vi "compare top countries window.vi"(4 "SA data":T1, 6 "Countries":string[](array[string]), 7 "Aggregate indexes":i32[](array[numeric]), 8 "Populations":i32[](array[numeric]), 9 "US data":T1, 10 "deaths CSV":string[][](array[string]), 11 "cases CSV":string[][](array[string])) -> ()   [LabVIEW 2019]
uses:
  <vilib>/Utility/config.llb/NI_LVConfig.lvlib
panel:
  in  "Tab Control":enum32{"Results", "Filter out"}(tab)
  in  "Include SA provinces":bool
  in  "How far back to look for rate of rise and fall (days)":u16=7
  out "Top cumulative deaths per M":string[](array[string])
  out "Top daily death rate per million ever":string[](array[string])
  out "Top rate of fall in deaths":string[](array[string]) caption="Top rate of fall in deaths (over last 7 days)"
  out "Top rate of rise in deaths (over last 14 days)":string[](array[string]) caption="Top rate of rise in deaths (over last 7 days)"
  out "Top new cases":string[](array[string])
  out "Top new deaths":string[](array[string])
  out "Top new cases per 1M":string[](array[string])
  out "Top new deaths per 1M":string[](array[string])
  in  "Include US states":bool
  in  "Include aggregates":bool
  in  "Aggregates":i32(listbox)
  in  "Remove Button":bool
  in  "Add Button":bool
  in  "Filter out":i32[](listbox)
  in  "Select Country":i32[](listbox)
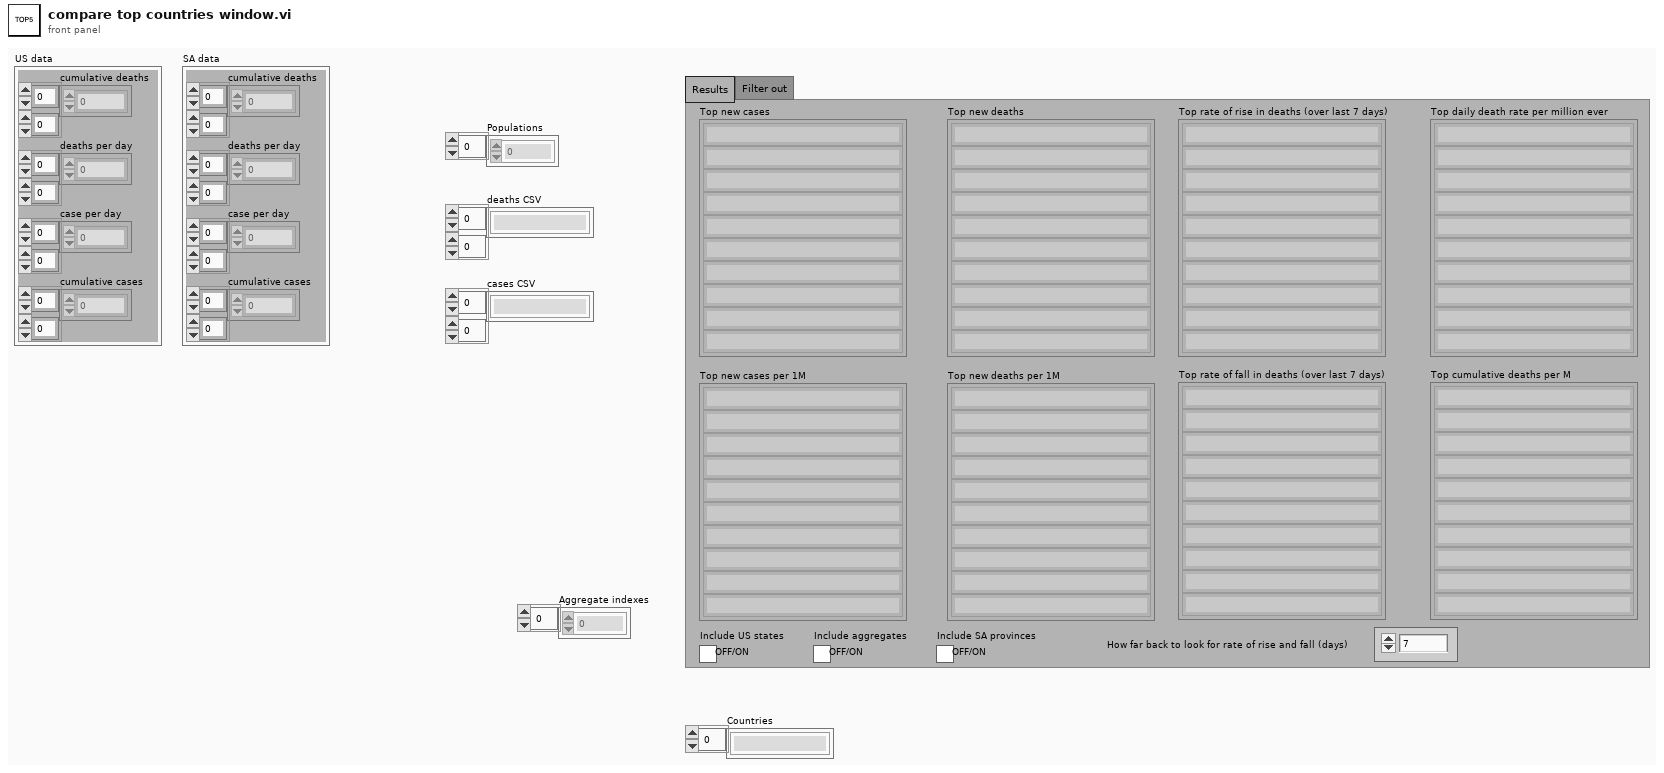
[diagram p1: front panel]
types:
  T1 = cluster{"cumulative deaths":i32[][], "deaths per day":i32[][], "case per day":i32[][], "cumulative cases":i32[][]}
  T2 = typedef "NI_LVConfig.lvlib/Config Data RefNum.ctl" = refnum<k1>
  T3 = cluster{"top new cases":cluster{"country index":i32[], "values":i32[]}, "top new deaths":cluster{"country index":i32[], "values":i32[]}, "top new cases per 1M":cluster{"country index":i32[], "values":dbl[]}, "top new deaths per 1M":cluster{"country index":i32[], "values":dbl[]}, "deaths dropped":cluster{"country index":i32[], "percentage change":dbl[]}, "deaths gained":cluster{"country index":i32[], "percentage change":dbl[]}, "highest deaths per day ever":cluster{"country index":i32[], "highest deaths per day":dbl[]}, "highest deaths":cluster{"country index":i32[], "highest deaths per day":dbl[]}}
  T4 = cluster{"country index":i32[], "percentage change":dbl[]}
  T5 = cluster{"country index":i32[], "highest deaths per day":dbl[]}
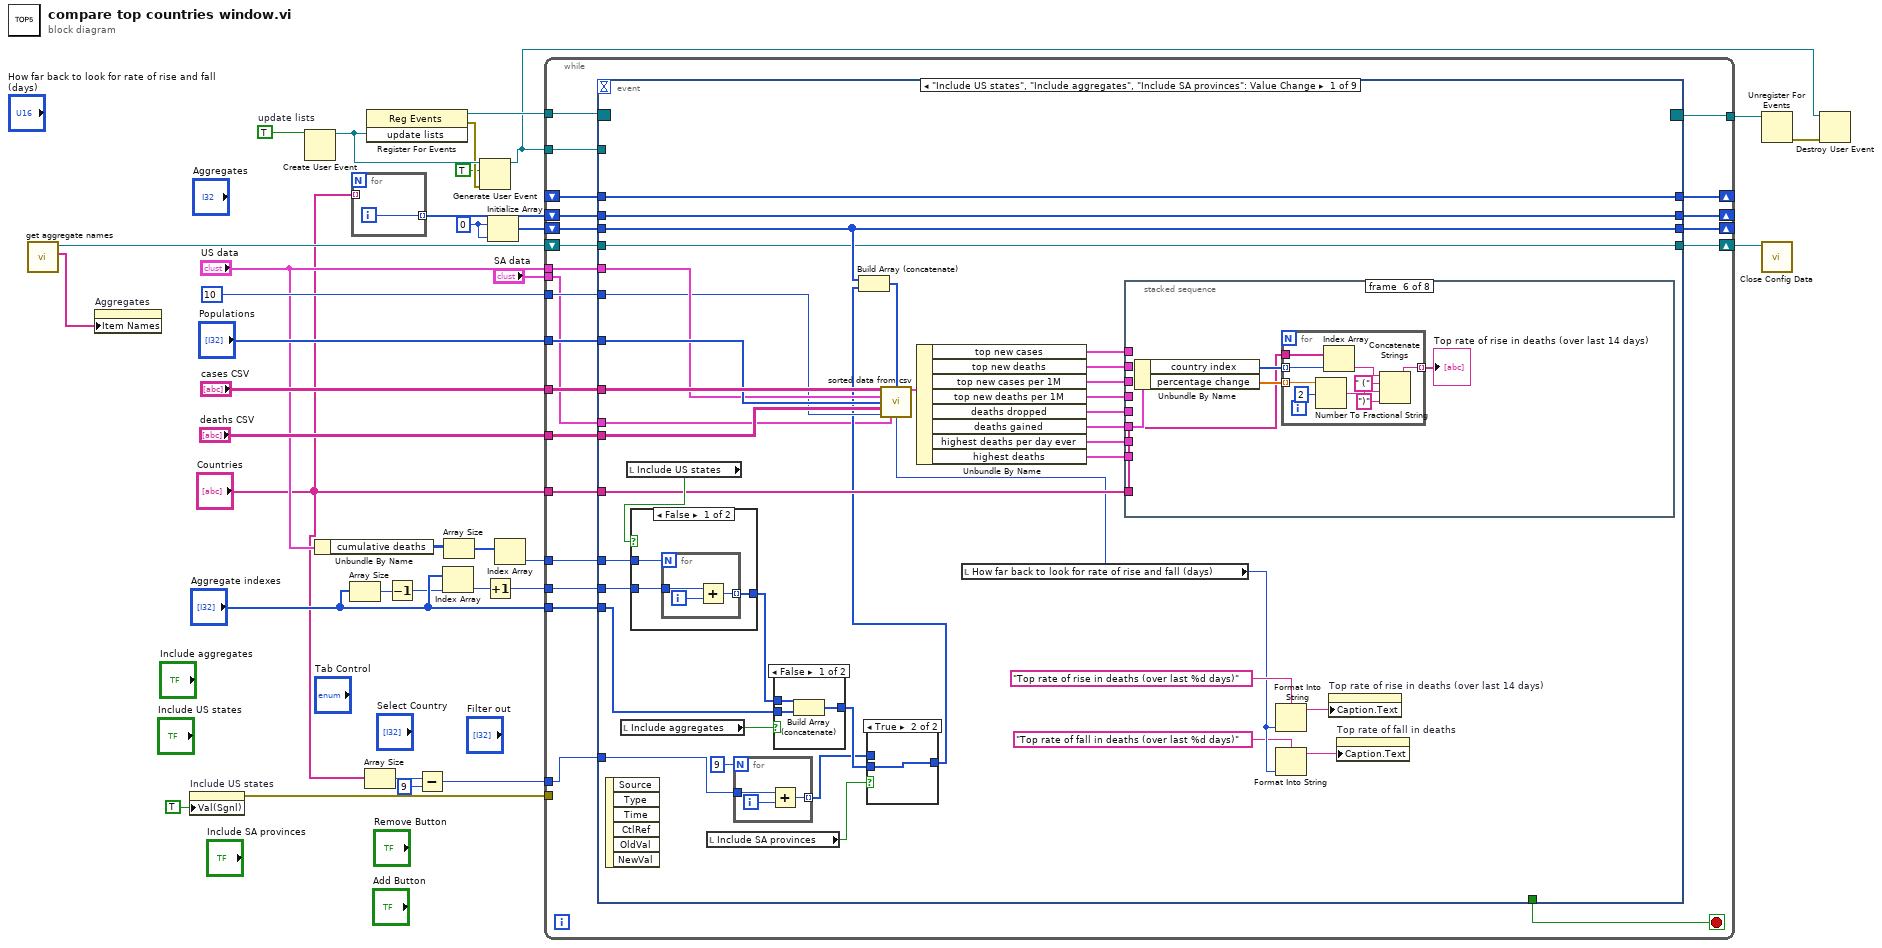
[diagram p0: block diagram]
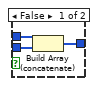
[diagram p2: hidden frame]
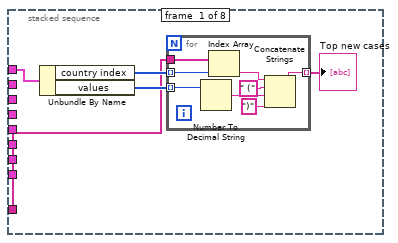
[diagram p3: hidden frame]
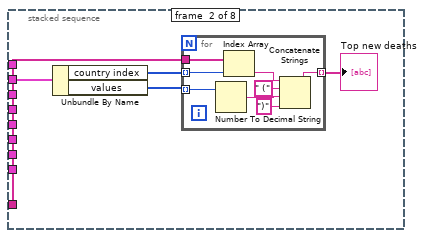
[diagram p4: hidden frame]
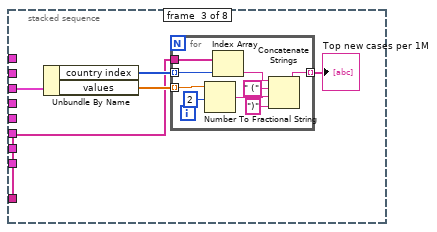
[diagram p5: hidden frame]
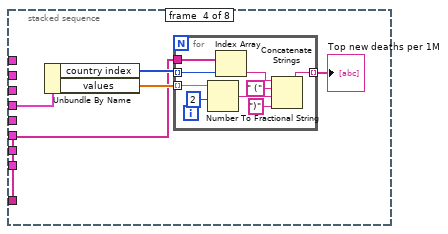
[diagram p6: hidden frame]
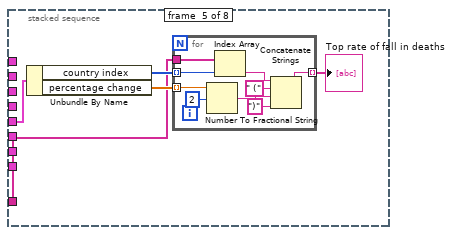
[diagram p7: hidden frame]
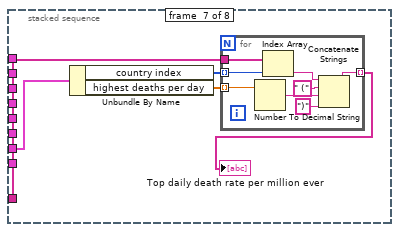
[diagram p8: hidden frame]
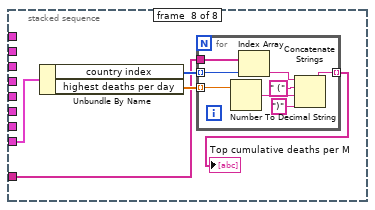
[diagram p9: hidden frame]
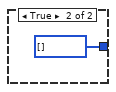
[diagram p10: hidden frame]
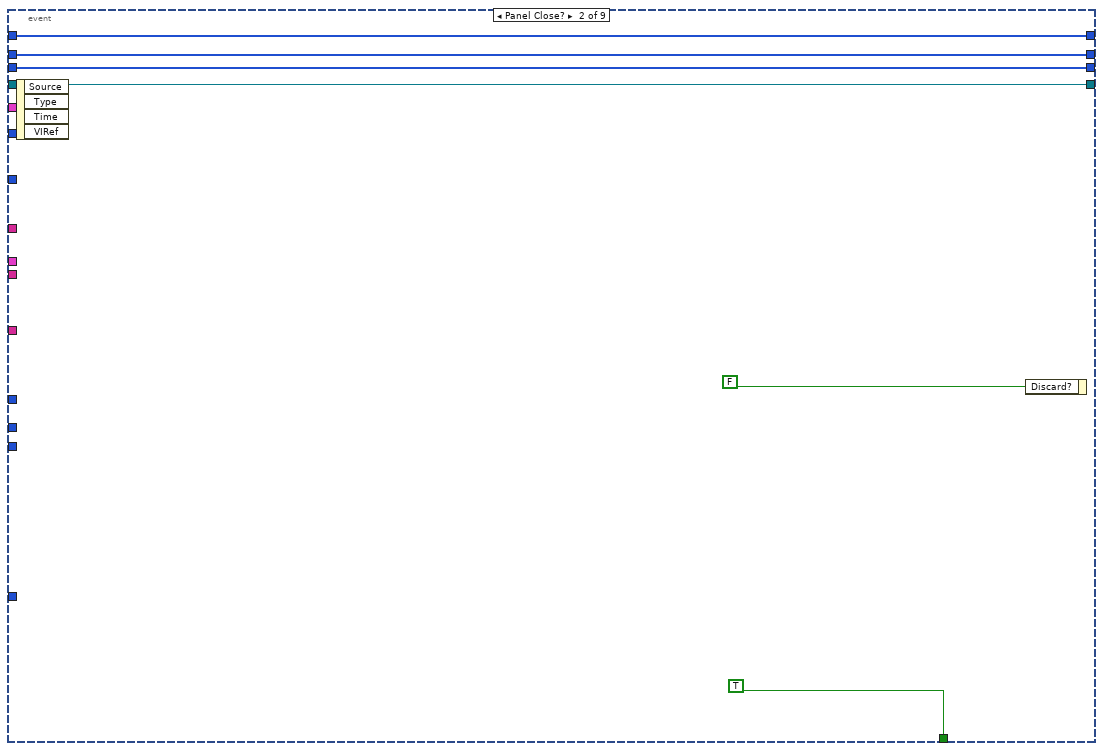
[diagram p12: hidden frame]
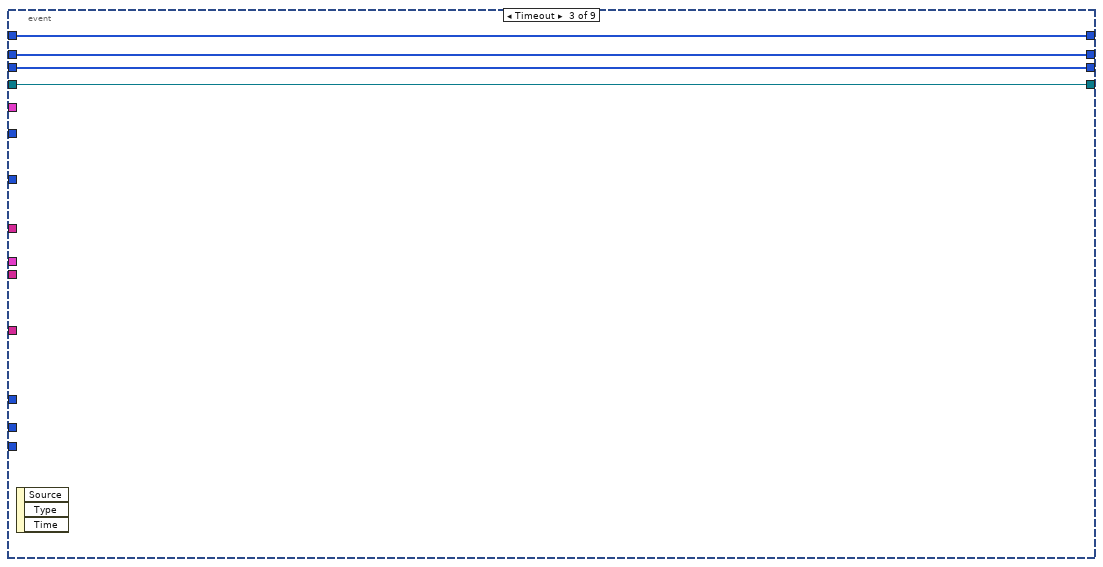
[diagram p13: hidden frame]
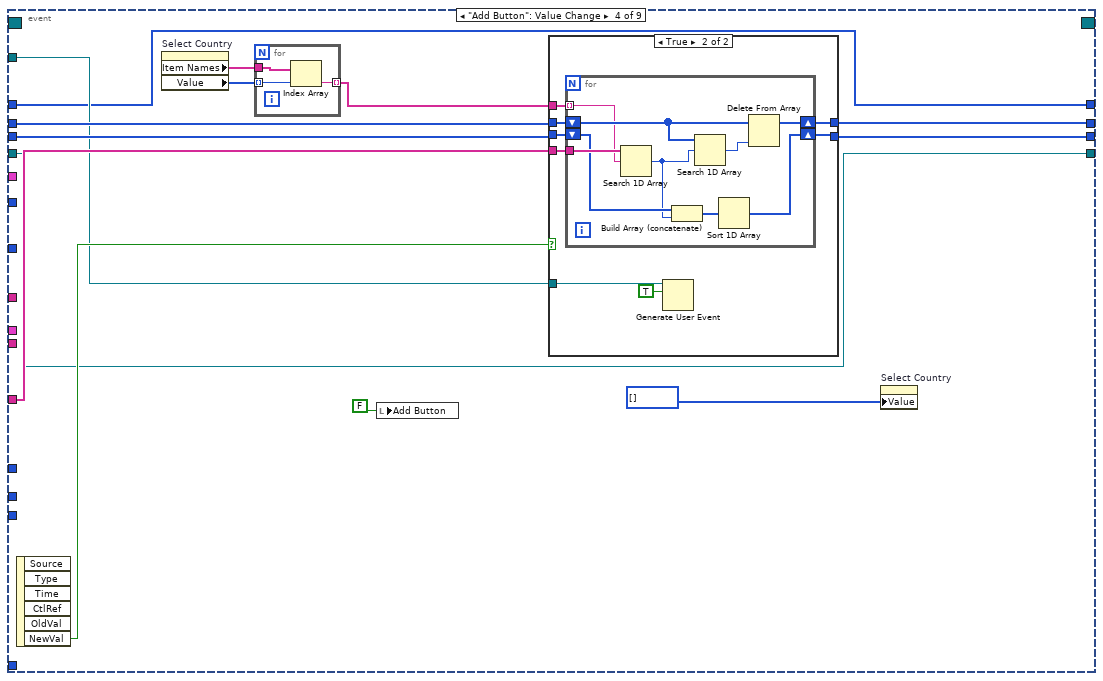
[diagram p14: hidden frame]
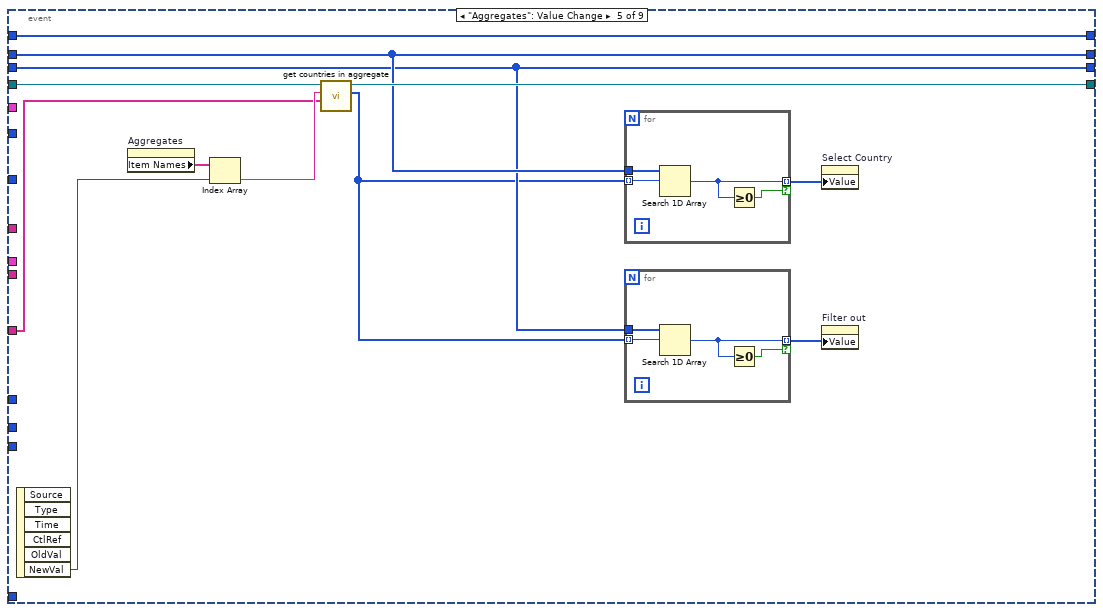
[diagram p16: hidden frame]
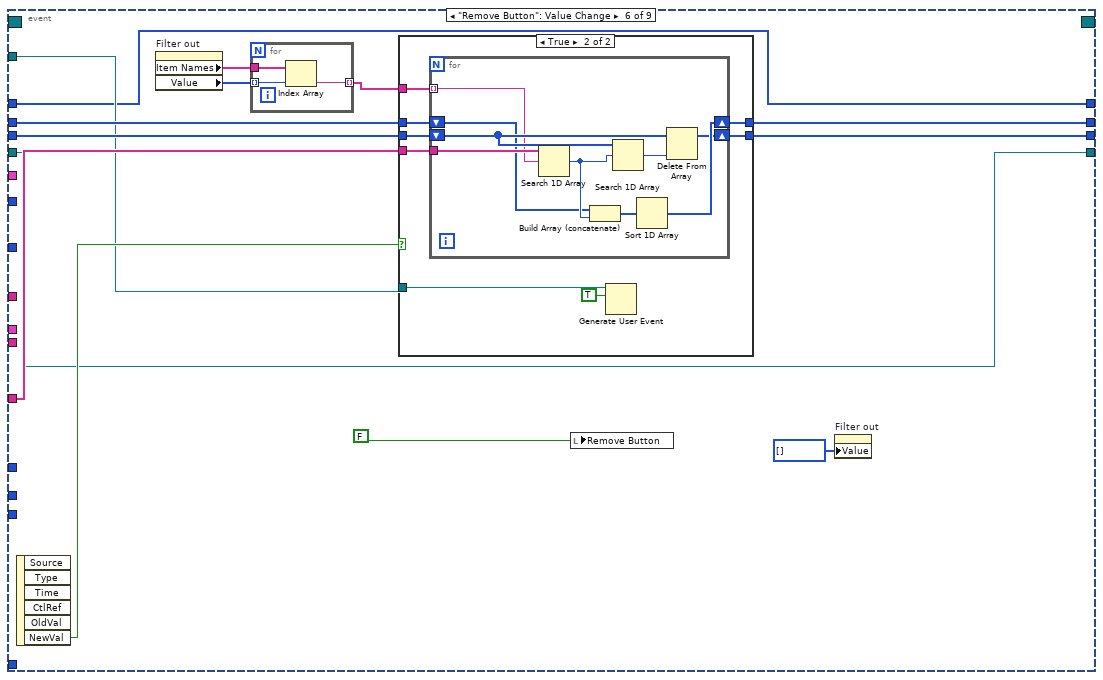
[diagram p17: hidden frame]
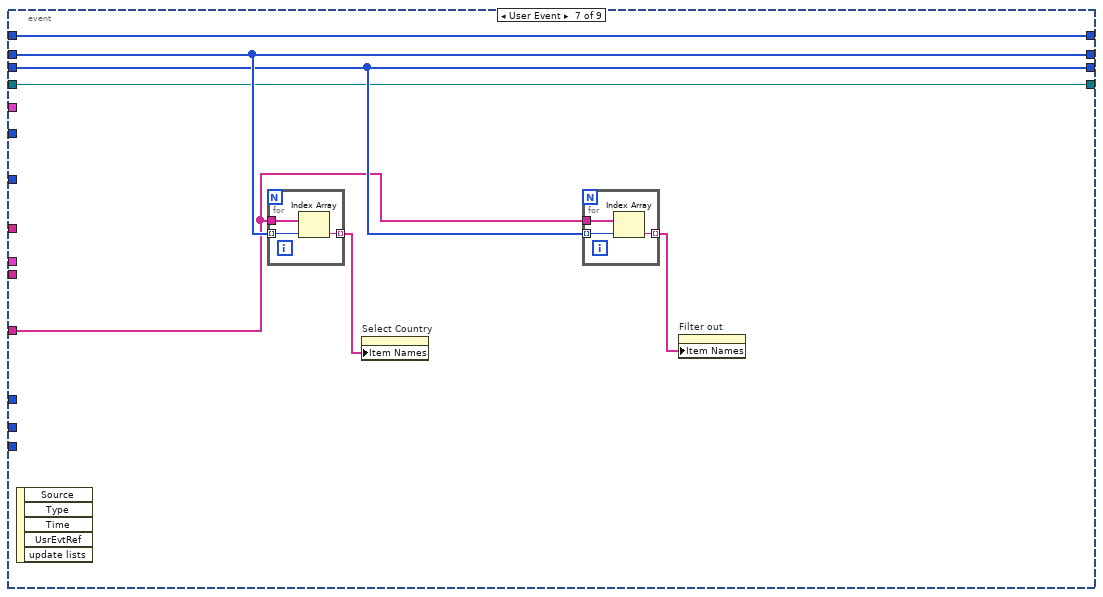
[diagram p19: hidden frame]
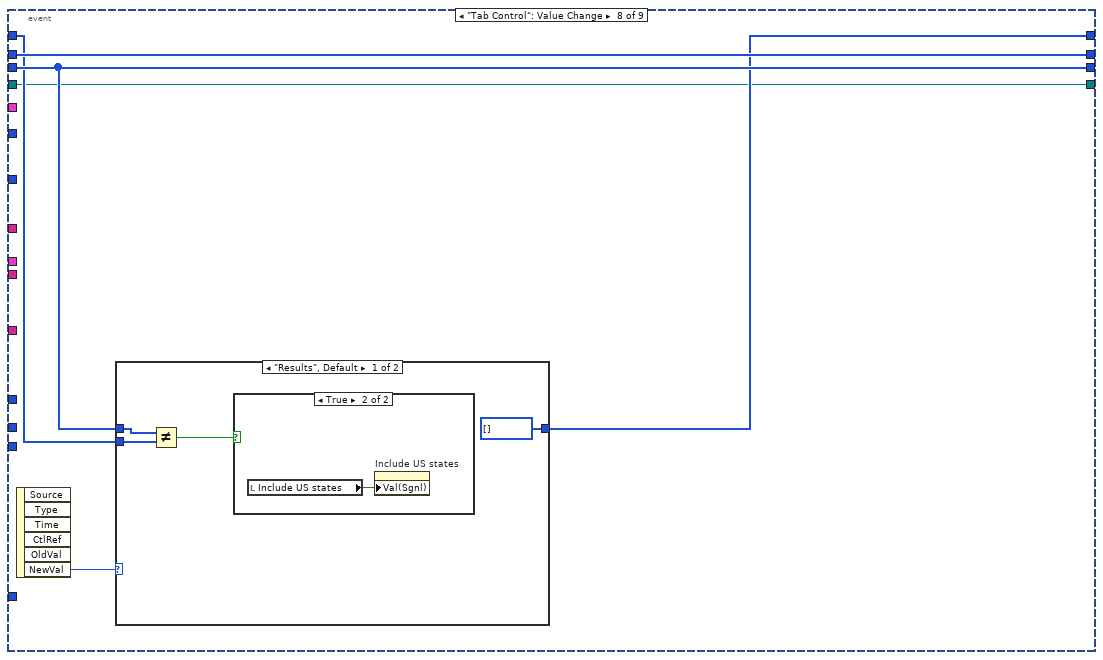
[diagram p20: hidden frame]
diagram:
  w19 = TRUE  # update lists
  w22 = 0
  n1 = call "get aggregate names.vi"() -> ("section names"=w8:string[], "Refnum out"=w7:T2)  [unwired: 10 in]
  n2 = property on="Aggregates" class="LstBox (strict)"("Item Names"=w8) -> ()  [unwired: 2 in, 2 out]
  n3 = property on="Include US states" class="Bool (strict)"("Val(Sgnl)"=TRUE ("Value (Signaling)")) -> (error out=w29:errorcluster)  [unwired: 2 in, 1 out]
  n4 = Create User Event(user event datatype=w19) -> (user event=w15:refnum<user-event>)  [unwired: 1 in, 1 out]
  n5 = Unbundle By Name("US data") -> ("cumulative deaths"=w27:i32[][])
  n6 = Array Size(array="Aggregate indexes") -> (size(s)=w10:i32)
  n7 = for {
    tunnel: "Countries" -> [_] mode=indexing
    tunnel: [w35] -> w20 mode=indexing
    i -> [w35]
  }
  n8 = Array Size(array="Countries") -> (size(s)=w4:i32)
  n9 = register-events(w15) -> (reference out=w18:refnum<event-registration>, error out=w13:errorcluster)  [unwired: 2 in]
  n10 = Decrement(x=w10) -> (x-1=w9:i32)
  n11 = Subtract(x=w4, y=9) -> (x-y=w2:i32)
  n12 = Index Array(array="Aggregate indexes", index=w9) -> (element=w24:i32)
  n13 = Array Size(array=w27) -> (size(s)=w26:i32[])
  n14 = Generate User Event(user event=w15, event data cluster=TRUE ("event data"), error in=w13) -> (user event out=w14:refnum<user-event>)  [unwired: 1 in, 1 out]
  n15 = Increment(x=w24) -> (x+1=w23:i32)
  n16 = Initialize Array(w22, w22) -> (w21:i32[])
  n17 = Index Array(array=w26) -> (element=w25:i32)  [unwired: 1 in]
  n18 = while {
    tunnel: "cases CSV" -> [w58]
    tunnel: "deaths CSV" -> [w57]
    tunnel: "Countries" -> [w56]
    tunnel: "Populations" -> [w55]
    tunnel: "US data" -> [w54]
    tunnel: 10 ("top selection") -> [w53]
    tunnel: w29 -> [_]
    tunnel: "Aggregate indexes" -> [w51]
    tunnel: w25 -> [w50]
    tunnel: w23 -> [w49]
    shift-right: [w47] -> _
    shift-left: w20 -> [w48]
    shift-right: [w45] -> _
    shift-left: w21 -> [w46]
    tunnel: w18 -> [w44]
    tunnel: w14 -> [w43]
    tunnel: [w42] -> w17
    shift-right: [w41] -> _
    shift-left: _ -> [w40]
    shift-right: [w38] -> w6
    shift-left: w7 -> [w39]
    tunnel: w2 -> [w37]
    tunnel: "SA data" -> [w36]
    stop <- w52 stop-if-true
    n19 = event shown="[0] \"Include US states\", \"Include aggregates\", \"Include SA provinces\": Value Change" {
      selector: w44 -> [_ _ _ _ _ _ _ _ _]
      dyn-events: [_ _ _ _ _ _ _ _ _] -> w42
      timeout: _ -> [_ _ _ _ _ _ _ _ _]
      tunnel: w58 -> [w96 _ _ _ _ _ _ _ _]
      tunnel: w57 -> [w95 _ _ _ _ _ _ _ _]
      tunnel: w56 -> [w78 _ _ w244 w275 w298 w329 _ _]
      tunnel: w55 -> [w94 _ _ _ _ _ _ _ _]
      tunnel: w54 -> [w93 _ _ _ _ _ _ _ _]
      tunnel: w53 -> [w92 _ _ _ _ _ _ _ _]
      tunnel: [_ TRUE _ _ _ _ _ _ _] -> w52
      tunnel: w51 -> [w90 _ _ _ _ _ _ _ _]
      tunnel: w50 -> [w87 _ _ _ _ _ _ _ _]
      tunnel: w49 -> [w86 _ _ _ _ _ _ _ _]
      tunnel: w48 -> [w85 w226 w232 w246 w274 w302 w331 w343 w354]
      tunnel: [w85 w226 w232 w243 w274 w300 w331 w343 w354] -> w47
      tunnel: w46 -> [w83 w225 w231 w245 w270 w301 w330 w341 w353]
      tunnel: [w83 w225 w231 w242 w270 w299 w330 w341 w353] -> w45
      tunnel: w43 -> [_ _ _ w240 _ w296 _ _ _]
      tunnel: [w82 w224 w230 w239 w280 w295 w326 w340 w352] -> w41
      tunnel: w40 -> [w82 w224 w230 w239 w280 w295 w326 w339 w352]
      tunnel: w39 -> [w81 w223 w229 w235 w279 w294 w325 w338 w351]
      tunnel: [w81 w223 w229 w235 w278 w294 w325 w338 w351] -> w38
      tunnel: w37 -> [w60 _ _ _ _ _ _ _ _]
      tunnel: w36 -> [w59 _ _ _ _ _ _ _ _]
      event "Include US states", "Include aggregates", "Include SA provinces": Value Change {
        n20 = event-data() -> ()  [unwired: 1 in, 6 out]
        n21 = local read "Include aggregates"() -> (w91:bool)
        n22 = local read "Include US states"() -> (w89:bool)
        n23 = case shown="False" w89 {
          tunnel: [w214 i32[] [] ("Aggregate indexes")] -> w88
          tunnel: w87 -> [w213 _]
          tunnel: w86 -> [w212 _]
          frame False {
            n24 = for {
              N: w213 -> [_]
              tunnel: [w217] -> w214 mode=indexing
              tunnel: w212 -> [w215]
              i -> [w216]
              n25 = Add(x=w215, y=w216) -> (x+y=w217:i32)
            }
          }
          frame True {
          }
        }
        n26 = local read "Include SA provinces"() -> (w64:bool)
        n27 = for {
          N: 9 -> [_]
          tunnel: [w99] -> w61 mode=indexing
          tunnel: w60 -> [w97]
          i -> [w98]
          n28 = Add(x=w97, y=w98) -> (x+y=w99:i32)
        }
        n29 = case shown="False" w91 {
          tunnel: w90 -> [w221 w222]
          tunnel: [w220 w222] -> w63
          tunnel: w88 -> [w219 _]
          frame False {
            n30 = Build Array (concatenate)(w219, w221) -> (w220:i32[])
          }
          frame True {
          }
        }
        n31 = case shown="True" w64 {
          tunnel: w63 -> [w102 w103]
          tunnel: [w101 w103] -> w65
          tunnel: w61 -> [w100 _]
          frame False {
            n32 = Build Array (concatenate)(w100, w102) -> (w101:i32[])
          }
          frame True {
          }
        }
        n33 = Build Array (concatenate)(w83, w65) -> (w84:i32[])
        n34 = local read "How far back to look for rate of rise and fall (days)"() -> (w69:u16)
        n35 = call "sorted data from csv.vi"("cases CSV"=w96, "filter out"=w84, "US data"=w93, "Populations"=w94, "deaths CSV"=w95, "top selection"=w92, "SA data"=w59, "period in days to check"=w69) -> ("ranked results"=w80:T3)  [unwired: 7 in]
        n36 = Unbundle By Name(w80) -> ("top new cases"=w79:cluster{"country index":i32[], "values":i32[]}, "top new deaths"=w77:cluster{"country index":i32[], "values":i32[]}, "top new cases per 1M"=w76:cluster{"country index":i32[], "values":dbl[]}, "top new deaths per 1M"=w75:cluster{"country index":i32[], "values":dbl[]}, "deaths dropped"=w74:T4, "deaths gained"=w73:T4, "highest deaths per day ever"=w72:T5, "highest deaths"=w71:T5)
        n37 = stacked-sequence {
          tunnel: w79 -> [w107 _ _ _ _ _ _ _]
          tunnel: w78 -> [w104 w119 w130 w144 w158 w172 w186 w199]
          tunnel: w77 -> [_ w118 _ _ _ _ _ _]
          tunnel: w76 -> [_ _ w131 _ _ _ _ _]
          tunnel: w75 -> [_ _ _ w145 _ _ _ _]
          tunnel: w74 -> [_ _ _ _ w159 _ _ _]
          tunnel: w73 -> [_ _ _ _ _ w173 _ _]
          tunnel: w72 -> [_ _ _ _ _ _ w187 _]
          tunnel: w71 -> [_ _ _ _ _ _ _ w203]
          frame #0 {
            n38 = Unbundle By Name(w107) -> ("country index"=w106:i32[], "values"=w105:i32[])
            n39 = for {
              tunnel: w106 -> [w109] mode=indexing
              tunnel: w104 -> [w116]
              tunnel: [w112] -> w108 mode=indexing
              tunnel: w105 -> [w110] mode=indexing
              n40 = Number To Decimal String(number=w110) -> (decimal integer string=w115:string)  [unwired: 1 in]
              n41 = Index Array(array=w116, index=w109) -> (element=w111:string)
              n42 = Concatenate Strings(w111, " (" ("string"), w115, ")" ("string")) -> (w112:string)
            }
            "Top new cases" <- w108
          }
          frame #1 {
            n43 = Unbundle By Name(w118) -> ("country index"=w121:i32[], "values"=w117:i32[])
            n44 = for {
              tunnel: w121 -> [w122] mode=indexing
              tunnel: w119 -> [w129]
              tunnel: [w125] -> w120 mode=indexing
              tunnel: w117 -> [w123] mode=indexing
              n45 = Number To Decimal String(number=w123) -> (decimal integer string=w128:string)  [unwired: 1 in]
              n46 = Index Array(array=w129, index=w122) -> (element=w124:string)
              n47 = Concatenate Strings(w124, " (" ("string"), w128, ")" ("string")) -> (w125:string)
            }
            "Top new deaths" <- w120
          }
          frame #2 {
            n48 = Unbundle By Name(w131) -> ("country index"=w133:i32[], "values"=w134:dbl[])
            n49 = for {
              tunnel: w133 -> [w135] mode=indexing
              tunnel: w130 -> [w143]
              tunnel: [w139] -> w132 mode=indexing
              tunnel: w134 -> [w137] mode=indexing
              n50 = Number To Fractional String(number=w137, precision (6)=i16 2) -> (F-format string=w142:string)  [unwired: 2 in]
              n51 = Index Array(array=w143, index=w135) -> (element=w138:string)
              n52 = Concatenate Strings(w138, " (" ("string"), w142, ")" ("string")) -> (w139:string)
            }
            "Top new cases per 1M" <- w132
          }
          frame #3 {
            n53 = Unbundle By Name(w145) -> ("country index"=w147:i32[], "values"=w148:dbl[])
            n54 = for {
              tunnel: w147 -> [w149] mode=indexing
              tunnel: w144 -> [w157]
              tunnel: [w153] -> w146 mode=indexing
              tunnel: w148 -> [w151] mode=indexing
              n55 = Number To Fractional String(number=w151, precision (6)=i16 2) -> (F-format string=w156:string)  [unwired: 2 in]
              n56 = Index Array(array=w157, index=w149) -> (element=w152:string)
              n57 = Concatenate Strings(w152, " (" ("string"), w156, ")" ("string")) -> (w153:string)
            }
            "Top new deaths per 1M" <- w146
          }
          frame #4 {
            n58 = Unbundle By Name(w159) -> ("country index"=w161:i32[], "percentage change"=w162:dbl[])
            n59 = for {
              tunnel: w161 -> [w163] mode=indexing
              tunnel: w158 -> [w171]
              tunnel: [w167] -> w160 mode=indexing
              tunnel: w162 -> [w165] mode=indexing
              n60 = Number To Fractional String(number=w165, precision (6)=i16 2) -> (F-format string=w170:string)  [unwired: 2 in]
              n61 = Index Array(array=w171, index=w163) -> (element=w166:string)
              n62 = Concatenate Strings(w166, " (" ("string"), w170, ")" ("string")) -> (w167:string)
            }
            "Top rate of fall in deaths" <- w160
          }
          frame #5 {
            n63 = Unbundle By Name(w173) -> ("country index"=w175:i32[], "percentage change"=w176:dbl[])
            n64 = for {
              tunnel: w175 -> [w177] mode=indexing
              tunnel: w172 -> [w185]
              tunnel: [w181] -> w174 mode=indexing
              tunnel: w176 -> [w179] mode=indexing
              n65 = Number To Fractional String(number=w179, precision (6)=i16 2) -> (F-format string=w184:string)  [unwired: 2 in]
              n66 = Index Array(array=w185, index=w177) -> (element=w180:string)
              n67 = Concatenate Strings(w180, " (" ("string"), w184, ")" ("string")) -> (w181:string)
            }
            "Top rate of rise in deaths (over last 14 days)" <- w174
          }
          frame #6 {
            n68 = Unbundle By Name(w187) -> ("country index"=w189:i32[], "highest deaths per day"=w188:dbl[])
            n69 = for {
              tunnel: w189 -> [w191] mode=indexing
              tunnel: w186 -> [w198]
              tunnel: [w194] -> w190 mode=indexing
              tunnel: w188 -> [w192] mode=indexing
              n70 = Number To Decimal String(number=w192) -> (decimal integer string=w197:string)  [unwired: 1 in]
              n71 = Index Array(array=w198, index=w191) -> (element=w193:string)
              n72 = Concatenate Strings(w193, " (" ("string"), w197, ")" ("string")) -> (w194:string)
            }
            "Top daily death rate per million ever" <- w190
          }
          frame #7 {
            n73 = Unbundle By Name(w203) -> ("country index"=w202:i32[], "highest deaths per day"=w201:dbl[])
            n74 = for {
              tunnel: w202 -> [w204] mode=indexing
              tunnel: w199 -> [w211]
              tunnel: [w207] -> w200 mode=indexing
              tunnel: w201 -> [w205] mode=indexing
              n75 = Number To Decimal String(number=w205) -> (decimal integer string=w210:string)  [unwired: 1 in]
              n76 = Index Array(array=w211, index=w204) -> (element=w206:string)
              n77 = Concatenate Strings(w206, " (" ("string"), w210, ")" ("string")) -> (w207:string)
            }
            "Top cumulative deaths per M" <- w200
          }
        }
        n78 = Format Into String(format string="Top rate of rise in deaths (over last %d days)", w69) -> (resulting string=w68:string)  [unwired: 2 in, 1 out]
        n79 = Format Into String(format string="Top rate of fall in deaths (over last %d days)", w69) -> (resulting string=w67:string)  [unwired: 2 in, 1 out]
        n80 = property on="Top rate of rise in deaths (over last 14 days)" class="Arr (strict)"("Caption.Text"=w68) -> ()  [unwired: 2 in, 2 out]
        n81 = property on="Top rate of fall in deaths" class="Arr (strict)"("Caption.Text"=w67) -> ()  [unwired: 2 in, 2 out]
      }
      event Panel Close? {
        n82 = event-data() -> ()  [unwired: 1 in, 4 out]
        n83 = event-data("Discard?"=FALSE) -> ()  [unwired: 1 in, 1 out]
      }
      event Timeout {
        n84 = event-data() -> ()  [unwired: 1 in, 3 out]
      }
      event "Add Button": Value Change {
        n85 = event-data() -> ("NewVal"=w241:bool)  [unwired: 1 in, 5 out]
        n86 = property on="Select Country" class="LstBox (strict)"() -> ("Item Names"=w237:string[], "Value"=w238:i32[])  [unwired: 2 in, 2 out]
        n87 = for {
          tunnel: w238 -> [w249] mode=indexing
          tunnel: w237 -> [w248]
          tunnel: [w247] -> w236 mode=indexing
          n88 = Index Array(array=w248, index=w249) -> (element=w247:string)
        }
        n89 = local write "Add Button"(FALSE ("Add Button")) -> ()
        n90 = case shown="True" w241 {
          tunnel: w246 -> [w251 w258]
          tunnel: w244 -> [_ w259]
          tunnel: [w251 w253] -> w243
          tunnel: w245 -> [w250 w257]
          tunnel: [w250 w254] -> w242
          tunnel: w240 -> [_ w256]
          tunnel: w236 -> [_ w252]
          frame False {
          }
          frame True {
            n91 = for {
              tunnel: w259 -> [w268]
              shift-right: [w262] -> w254
              shift-left: w257 -> [w265]
              shift-right: [w261] -> w253
              shift-left: w258 -> [w266]
              tunnel: w252 -> [w260] mode=indexing
              n92 = Search 1D Array(1D array=w268, element=w260) -> (index of element=w264:i32)  [unwired: 1 in]
              n93 = Build Array (concatenate)(w265, w264) -> (w263:i32[])
              n94 = Search 1D Array(1D array=w266, element=w264) -> (index of element=w267:i32)  [unwired: 1 in]
              n95 = Sort 1D Array(array=w263) -> (sorted array=w262:i32[])
              n96 = Delete From Array(array=w266, index=w267) -> (array with subset deleted=w261:i32[])  [unwired: 1 in, 1 out]
            }
            n97 = Generate User Event(user event=w256, event data cluster=TRUE ("event data")) -> ()  [unwired: 2 in, 2 out]
          }
        }
        n98 = property on="Select Country" class="LstBox (strict)"("Value"=i32[] [] ("Select Country")) -> ()  [unwired: 2 in, 2 out]
      }
      event "Aggregates": Value Change {
        n99 = event-data() -> ("NewVal"=w272:i32)  [unwired: 1 in, 5 out]
        n100 = property on="Aggregates" class="LstBox (strict)"() -> ("Item Names"=w277:string[])  [unwired: 2 in, 2 out]
        n101 = Index Array(array=w277, index=w272) -> (element=w276:string)
        n102 = call "get countries in aggregate.vi"("countries"=w275, "aggregate name"=w276, "Refnum in"=w279) -> ("country indexes"=w269:i32[], "Refnum out"=w278:T2)  [unwired: 7 in]
        n103 = for {
          tunnel: w269 -> [w288] mode=indexing
          tunnel: w274 -> [w287]
          tunnel: [w286] -> w273 mode=indexing if=w285
          n104 = Search 1D Array(1D array=w287, element=w288) -> (index of element=w286:i32)  [unwired: 1 in]
          n105 = Greater Or Equal To 0?(x=w286) -> (x >= 0?=w285:bool)
        }
        n106 = for {
          tunnel: w269 -> [w284] mode=indexing
          tunnel: w270 -> [w283]
          tunnel: [w282] -> w271 mode=indexing if=w281
          n107 = Search 1D Array(1D array=w283, element=w284) -> (index of element=w282:i32)  [unwired: 1 in]
          n108 = Greater Or Equal To 0?(x=w282) -> (x >= 0?=w281:bool)
        }
        n109 = property on="Select Country" class="LstBox (strict)"("Value"=w273) -> ()  [unwired: 2 in, 2 out]
        n110 = property on="Filter out" class="LstBox (strict)"("Value"=w271) -> ()  [unwired: 2 in, 2 out]
      }
      event "Remove Button": Value Change {
        n111 = event-data() -> ("NewVal"=w297:bool)  [unwired: 1 in, 5 out]
        n112 = property on="Filter out" class="LstBox (strict)"() -> ("Item Names"=w291:string[], "Value"=w290:i32[])  [unwired: 2 in, 2 out]
        n113 = for {
          tunnel: w291 -> [w305]
          tunnel: w290 -> [w304] mode=indexing
          tunnel: [w303] -> w289 mode=indexing
          n114 = Index Array(array=w305, index=w304) -> (element=w303:string)
        }
        n115 = case shown="True" w297 {
          tunnel: w302 -> [w307 w313]
          tunnel: w298 -> [_ w315]
          tunnel: [w307 w309] -> w300
          tunnel: w301 -> [w306 w314]
          tunnel: [w306 w308] -> w299
          tunnel: w296 -> [_ w312]
          tunnel: w289 -> [_ w310]
          frame False {
          }
          frame True {
            n116 = for {
              tunnel: w315 -> [w324]
              tunnel: w310 -> [w318] mode=indexing
              shift-right: [w317] -> w309
              shift-left: w313 -> [w319]
              shift-right: [w316] -> w308
              shift-left: w314 -> [w320]
              n117 = Search 1D Array(1D array=w324, element=w318) -> (index of element=w322:i32)  [unwired: 1 in]
              n118 = Build Array (concatenate)(w319, w322) -> (w321:i32[])
              n119 = Search 1D Array(1D array=w320, element=w322) -> (index of element=w323:i32)  [unwired: 1 in]
              n120 = Sort 1D Array(array=w321) -> (sorted array=w317:i32[])
              n121 = Delete From Array(array=w320, index=w323) -> (array with subset deleted=w316:i32[])  [unwired: 1 in, 1 out]
            }
            n122 = Generate User Event(user event=w312, event data cluster=TRUE ("event data")) -> ()  [unwired: 2 in, 2 out]
          }
        }
        n123 = local write "Remove Button"(FALSE ("Remove Button")) -> ()
        n124 = property on="Filter out" class="LstBox (strict)"("Value"=i32[] [] ("Filter out")) -> ()  [unwired: 2 in, 2 out]
      }
      event User Event {
        n125 = event-data() -> ()  [unwired: 1 in, 5 out]
        n126 = for {
          tunnel: w331 -> [w336] mode=indexing
          tunnel: w329 -> [w337]
          tunnel: [w335] -> w328 mode=indexing
          n127 = Index Array(array=w337, index=w336) -> (element=w335:string)
        }
        n128 = property on="Select Country" class="LstBox (strict)"("Item Names"=w328) -> ()  [unwired: 2 in, 2 out]
        n129 = for {
          tunnel: w330 -> [w333] mode=indexing
          tunnel: w329 -> [w334]
          tunnel: [w332] -> w327 mode=indexing
          n130 = Index Array(array=w334, index=w333) -> (element=w332:string)
        }
        n131 = property on="Filter out" class="LstBox (strict)"("Item Names"=w327) -> ()  [unwired: 2 in, 2 out]
      }
      event "Tab Control": Value Change {
        n132 = event-data() -> ("NewVal"=w342:enum32{"Results", "Filter out"})  [unwired: 1 in, 5 out]
        n133 = case shown="\"Results\", Default" w342 {
          tunnel: w341 -> [w347 w349]
          tunnel: [i32[] [] w349] -> w340
          tunnel: w339 -> [w346 _]
          frame "Results", Default {
            n134 = Not Equal?(x=w347, y=w346) -> (x != y?=w344:bool)
            n135 = case shown="True" w344 {
              frame False {
              }
              frame True {
                n136 = local read "Include US states"() -> (w348:bool)
                n137 = property on="Include US states" class="Bool (strict)"("Val(Sgnl)"=w348) -> ()  [unwired: 2 in, 2 out]
              }
            }
          }
          frame "Filter out" {
          }
        }
      }
      event "How far back to look for rate of rise and fall (days)": Value Change {
        n138 = event-data() -> ()  [unwired: 1 in, 6 out]
        n139 = local read "Include US states"() -> (w350:bool)
        n140 = property on="Include US states" class="Bool (strict)"("Val(Sgnl)"=w350) -> ()  [unwired: 2 in, 2 out]
      }
    }
  }
  n141 = Unregister For Events(event registration refnum=w17) -> (error out=w16:errorcluster)  [unwired: 1 in]
  n142 = call <vilib>:"Close Config Data.vi"("refnum"=w6) -> ()  [unwired: 9 in, 2 out]
  n143 = Destroy User Event(user event=w14, error in=w16) -> ()  [unwired: 1 out]
